vi "GetAutoIndices.vi"() -> (1 "LLL Routine Index":u16, 2 "LRL Routine Index":u16, 3 "RLR Routine Index":u16, 4 "RRR Routine Index":u16)   [LabVIEW 2017]
uses:
  <vilib>/Rock Robotics/Network Tables/NT Read Number.vi
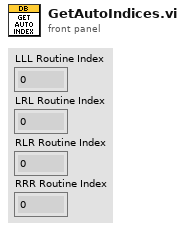
[diagram p1: front panel]
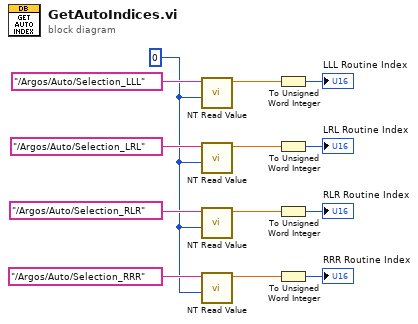
[diagram p0: block diagram]
diagram:
  w1 = u16 0 ("LLL Routine Index")
  n1 = call-poly <vilib>:"NT Read Value.vi"("Default Value"=w1, "Name"="/Argos/Auto/Selection_LLL") -> ("Numeric"=w9:dbl)  [unwired: 8 in, 1 out]
  n2 = call-poly <vilib>:"NT Read Value.vi"("Default Value"=w1, "Name"="/Argos/Auto/Selection_LRL") -> ("Numeric"=w6:dbl)  [unwired: 8 in, 1 out]
  n3 = call-poly <vilib>:"NT Read Value.vi"("Default Value"=w1, "Name"="/Argos/Auto/Selection_RLR") -> ("Numeric"=w7:dbl)  [unwired: 8 in, 1 out]
  n4 = call-poly <vilib>:"NT Read Value.vi"("Default Value"=w1, "Name"="/Argos/Auto/Selection_RRR") -> ("Numeric"=w8:dbl)  [unwired: 8 in, 1 out]
  n5 = To Unsigned Word Integer(number=w9) -> (unsigned 16bit integer=→"LLL Routine Index":u16)
  n6 = To Unsigned Word Integer(number=w6) -> (unsigned 16bit integer=→"LRL Routine Index":u16)
  n7 = To Unsigned Word Integer(number=w7) -> (unsigned 16bit integer=→"RLR Routine Index":u16)
  n8 = To Unsigned Word Integer(number=w8) -> (unsigned 16bit integer=→"RRR Routine Index":u16)
